vi "Read Delimiters.vi"(8 "Error In":errorcluster, 11 "Token In":refnum<class "Abstract.lvclass">) -> (0 "Error Out":errorcluster, 2 "Delimiters":cluster{"Close":string, "Open":string}, 3 "Token Out":refnum<class "Abstract.lvclass">)   [LabVIEW 2018, in "Toolkit.lvlib" / "Tokens.lvlib" / "Abstract.lvclass"]
uses:
  Abstract.lvclass
  Abstract.lvclass/Abstract.ctl
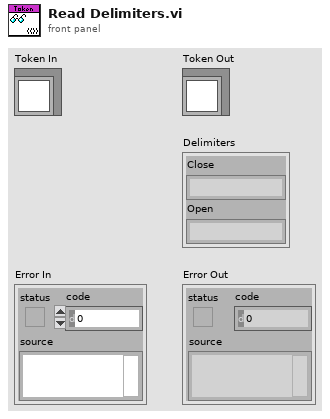
[diagram p1: front panel]
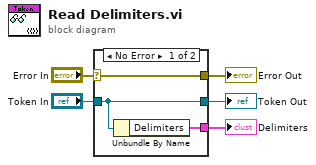
[diagram p0: block diagram]
diagram:
  n1 = case shown="No Error" "Error In" {
    selector: "Error In" -> [w8 w10]
    tunnel: [w8 w10] -> w4
    tunnel: [w7 w9] -> w2
    tunnel: "Token In" -> [w7 w9]
    tunnel: [w6 _] -> w1
    frame No Error {
      n2 = Unbundle By Name(w7) -> ("Delimiters"=w6:cluster{"Close":string, "Open":string})
    }
    frame Error {
    }
  }
  "Error Out" <- w4
  "Token Out" <- w2
  "Delimiters" <- w1
